vi "Read Radio Button Text.vi"(8 "error in":errorcluster, 11 "Radio Button Reference in":refnum<vi>) -> (0 "error out":errorcluster, 1 "Value":string[](array[string]), 2 "Interpret As Unicode":bool, 3 "Radio Button Reference out":refnum<vi>)   [LabVIEW 2020, in "G-Unicode.lvlib"]
uses:
  G-Unicode.lvlib
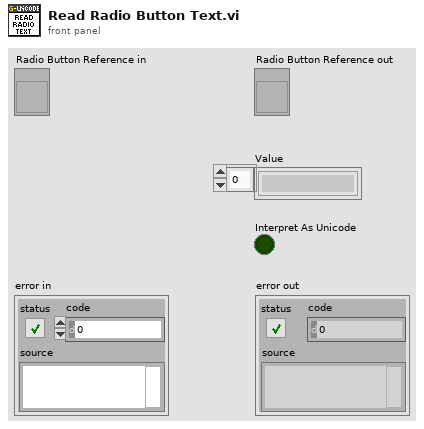
[diagram p1: front panel]
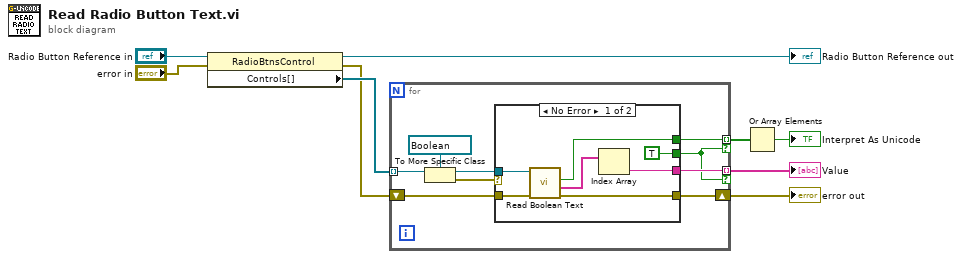
[diagram p0: block diagram]
diagram:
  n1 = property class="RadioBtnsControl"(reference="Radio Button Reference in", error in="error in") -> (reference out=→"Radio Button Reference out":refnum<vi>, error out=w2:errorcluster, "Controls[]"=w6:refnum<vi>[])
  n2 = for {
    tunnel: w6 -> [w15] mode=indexing
    tunnel: [w14] -> w5 mode=indexing if=w12
    tunnel: [w13] -> w4 mode=indexing if=w12
    shift-right: [w11] -> w1
    shift-left: w2 -> [w10]
    n3 = To More Specific Class(target class=refnum<vi> refnum ("Boolean Reference in"), reference=w15) -> (specific class reference=w16:refnum<vi>, error out=w17:errorcluster)  [unwired: 1 in]
    n4 = case shown="No Error" w17 {
      tunnel: w16 -> [w25 _]
      tunnel: w10 -> [w19 w26]
      tunnel: [w24 w26] -> w11
      tunnel: [w22 _] -> w14
      tunnel: [w21 _] -> w13
      tunnel: [TRUE _] -> w12
      frame No Error {
        n5 = call "Read Boolean Text.vi"("error in"=w19, "Boolean Reference in"=w25) -> ("error out"=w24:errorcluster, "Value"=w23:string[], "Interpret As Unicode"=w21:bool)  [unwired: 6 in, 1 out]
        n6 = Index Array(array=w23) -> (element=w22:string)  [unwired: 1 in]
      }
      frame Error {
      }
    }
  }
  "error out" <- w1
  "Value" <- w5
  n7 = Or Array Elements(Boolean array=w4) -> (logical OR=→"Interpret As Unicode":bool)
